vi "MenuItem Event Callback.vi"(4 "evNotifyIcon":refnum<user-event>, 5 "Event Data":cluster{"sender":refnum<k24>, "e":refnum<k24>}, 6 "Control Ref":refnum<k24>, 7 "Event Common Data":T1) -> ()   [LabVIEW 2017, in "NotifyIcon.lvclass"]
doc: "This is the Callback VI that gets called whenever the user clicks on a MenuItem in the Context Menu associated with the Notification Icon.\n\n\nStinus Olsen\nCIM Industrial Systems A/S\n22. Feb. 2011 15:04\nmailto: seo@cim.as"
uses:
  NotifyIcon.lvclass
  System.Windows.Forms
  Public/Controls/Notify Event.ctl
  Public/Controls/Notify Event Type.ctl
panel:
  # "This VI belongs to the NotifyIcon Toolset. \nA toolset that makes it easy to create, control and manipulate a notification icon in the notification area of the Windows taskbar.\nThe toolset requires Microsoft .NET framework 2.0\n\n\nNOTICE -- YOU MUST LEAVE THIS NOTICE IN PLACE.  PER THE TERMS OF THE LICENSE BELOW, YOU MAY SUBLICENSE THIS SOFTWARE \nIN ANY WAY THAT DOES NOT CONFLICT WITH THIS LICENSE.\n\n### BSD License (http://www.opensource.org/licenses/bsd-license.php) Begin ###\n \nCopyright (c) 2011, Stinus Olsen <seo@cim.as>\n\nAll rights reserved.\n\nRedistribution and use in source and binary forms, with or without modification, are permitted provided that the following conditions are met:\n\n    * Redistributions of source code must retain the above copyright notice, this list of conditions and the following disclaimer.\n    * Redistributions in binary form must reproduce the above copyright notice, this list of conditions and the following disclaimer in the \n       documentation and/or other materials provided with the distribution.\n    * Neither the name of CIM Industrial Systems nor the names of its contributors may be used to endorse or promote products derived \n       from this software without specific prior written permission.\n\nTHIS SOFTWARE IS PROVIDED BY THE COPYRIGHT HOLDERS AND CONTRIBUTORS \"AS IS\" AND ANY EXPRESS OR IMPLIED WARRANTIES, \nINCLUDING, BUT NOT LIMITED TO, THE IMPLIED WARRANTIES OF MERCHANTABILITY AND FITNESS FOR A PARTICULAR PURPOSE ARE \nDISCLAIMED. IN NO EVENT SHALL THE COPYRIGHT OWNER OR CONTRIBUTORS BE LIABLE FOR ANY DIRECT, INDIRECT, INCIDENTAL,\n SPECIAL, EXEMPLARY, OR CONSEQUENTIAL DAMAGES (INCLUDING, BUT NOT LIMITED TO, PROCUREMENT OF SUBSTITUTE GOODS OR \nSERVICES; LOSS OF USE, DATA, OR PROFITS; OR BUSINESS INTERRUPTION) HOWEVER CAUSED AND ON ANY THEORY OF LIABILITY, \nWHETHER IN CONTRACT, STRICT LIABILITY, OR TORT (INCLUDING NEGLIGENCE OR OTHERWISE) ARISING IN ANY WAY OUT OF THE USE \nOF THIS SOFTWARE, EVEN IF ADVISED OF THE POSSIBILITY OF SUCH DAMAGE.\n\n### BSD License End ###"
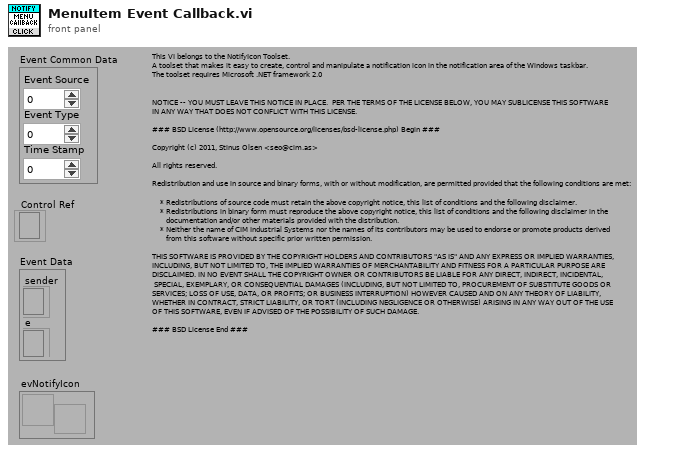
[diagram p1: front panel]
types:
  T1 = cluster{"Event Source":i32, "Event Type":u32, "Time Stamp":u32}
  T2 = typedef "NotifyIcon.lvclass/Notify Event.ctl" = cluster{"Type":T3, "Tag":string}
  T3 = typedef "NotifyIcon.lvclass/Notify Event Type.ctl" = enum16{"<Invalid Event>", "Tray Icon Click", "Tray Icon DoubleClick", "BalloonTip Shown", "BalloonTip Clicked", "BalloonTip Closed", "Menu Item Clicked"}
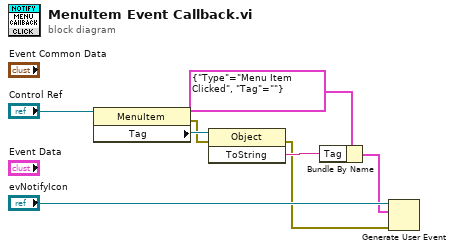
[diagram p0: block diagram]
diagram:
  n1 = property class="MenuItem"(reference="Control Ref") -> (error out=w1:errorcluster, "Tag"=w6:refnum<k24>)  [unwired: 1 in, 1 out]
  n2 = invoke class="Object" method="ToString"(reference=w6, error in=w1) -> (error out=w2:errorcluster, "ToString"=w4:string)  [unwired: 1 in, 1 out]
  n3 = Bundle By Name(cluster=T2 {"Type"=enum."Menu Item Clicked", "Tag"=""} ("event data"), "Tag"=w4) -> (w3:T2)
  n4 = Generate User Event(user event="evNotifyIcon", event data cluster=w3, error in=w2) -> ()  [unwired: 1 in, 2 out]
